vi "formal - Copy (2).vi"() -> ()   [LabVIEW 2011]
uses:
  <vilib>/DAQmx/read.llb/DAQmx Read (Analog 1D Wfm NChan NSamp).vi
  <vilib>/DAQmx/configure/timing.llb/DAQmx Timing (Sample Clock).vi
  <vilib>/DAQmx/miscellaneous.llb/DAQmx Fill In Error Info.vi
  C:/Program Files (x86)/National Instruments/LabVIEW 2011/resource/objmgr/daqmx.rc
  <vilib>/Analysis/NI_AALBase.lvlib
panel:
  out "Channel Name Array":string[](array[string])
  in  "index (col)":i32
  in  "voltage excitation source 2":i32(ring)=10200 items=["Internal"=10200, "External"=10167, "None"=10230]
  out "Config Array":T1(array[cluster])=[{[], "Voltage_cluster"={0.0, 0.0, 0.0, 0.0, TRUE, 0.0, 0.0}, "Strain_cluster"={0.0, 0.0, 0.0, 0.0, TRUE, 0.0, 0.0, 0.0, 0.0, ""}}, {[], "Voltage_cluster"={0.0, 0.0, 0.0, 0.0, TRUE, 0.0, 0.0}, "Strain_cluster"={0.0, 0.0, 0.0, 0.0, TRUE, 0.0, 0.0, 0.0, 0.0, ""}}, {[], "Voltage_cluster"={0.0, 0.0, 0.0, 0.0, TRUE, 0.0, 0.0}, "Strain_cluster"={0.0, 0.0, 0.0, 0.0, TRUE, 0.0, 0.0, 0.0, 0.0, ""}}, {[], "Voltage_cluster"={0.0, 0.0, 0.0, 0.0, TRUE, 0.0, 0.0}, "Strain_cluster"={0.0, 0.0, 0.0, 0.0, TRUE, 0.0, 0.0, 0.0, 0.0, ""}}, {[], "Voltage_cluster"={0.0, 0.0, 0.0, 0.0, TRUE, 0.0, 0.0}, "Strain_cluster"={0.0, 0.0, 0.0, 0.0, TRUE, 0.0, 0.0, 0.0, 0.0, ""}}, {[], "Voltage_cluster"={0.0, 0.0, 0.0, 0.0, TRUE, 0.0, 0.0}, "Strain_cluster"={0.0, 0.0, 0.0, 0.0, TRUE, 0.0, 0.0, 0.0, 0.0, ""}}, {[], "Voltage_cluster"={0.0, 0.0, 0.0, 0.0, TRUE, 0.0, 0.0}, "Strain_cluster"={0.0, 0.0, 0.0, 0.0, TRUE, 0.0, 0.0, 0.0, 0.0, ""}}, {[], "Voltage_cluster"={0.0, 0.0, 0.0, 0.0, TRUE, 0.0, 0.0}, "Strain_cluster"={0.0, 0.0, 0.0, 0.0, TRUE, 0.0, 0.0, 0.0, 0.0, ""}}]
  out "LVM result file path":path
  in  "Tab Control":T2(tab)
  out "Utility Usage Array":cluster{bool, string}[][](array[cluster])=[[{TRUE, "hjk"}, {FALSE, ""}, {FALSE, ""}, {FALSE, ""}], [{TRUE, "hjk"}, {FALSE, ""}, {FALSE, ""}, {FALSE, ""}], [{FALSE, ""}, {FALSE, ""}, {FALSE, ""}, {FALSE, ""}], [{FALSE, ""}, {FALSE, ""}, {FALSE, ""}, {FALSE, ""}], [{FALSE, ""}, {FALSE, ""}, {FALSE, ""}, {FALSE, ""}], [{FALSE, ""}, {FALSE, ""}, {FALSE, ""}, {FALSE, ""}], [{FALSE, ""}, {FALSE, ""}, {FALSE, ""}, {FALSE, ""}], [{FALSE, ""}, {FALSE, ""}, {FALSE, ""}, {FALSE, ""}]]
  in  "SXCI Chassis Name":string="/SC1"
  in  "Config File Path":path=path "M:/github/DAQP/xml_temp.xml"
  in  "Task Name":refnum<k21>="new Task"
  in  "Record File Path":string="trial_newnew"
  in  "error in":errorcluster
  in  "custom scale name":tag="linear1"
  in  "voltage excitation source":i32(ring)=10200 items=["Internal"=10200, "External"=10167, "None"=10230]
  in  "error out":errorcluster
  in  "sample rate":dbl=1000.0
  in  "number of samples per channel (buffer size)":i32=10000000
  in  "number of samples per channel":i32=100
  in  "Start DAQ":bool
  out "Result Array":dbl[](graph) caption="Voltage based transducer Reading"
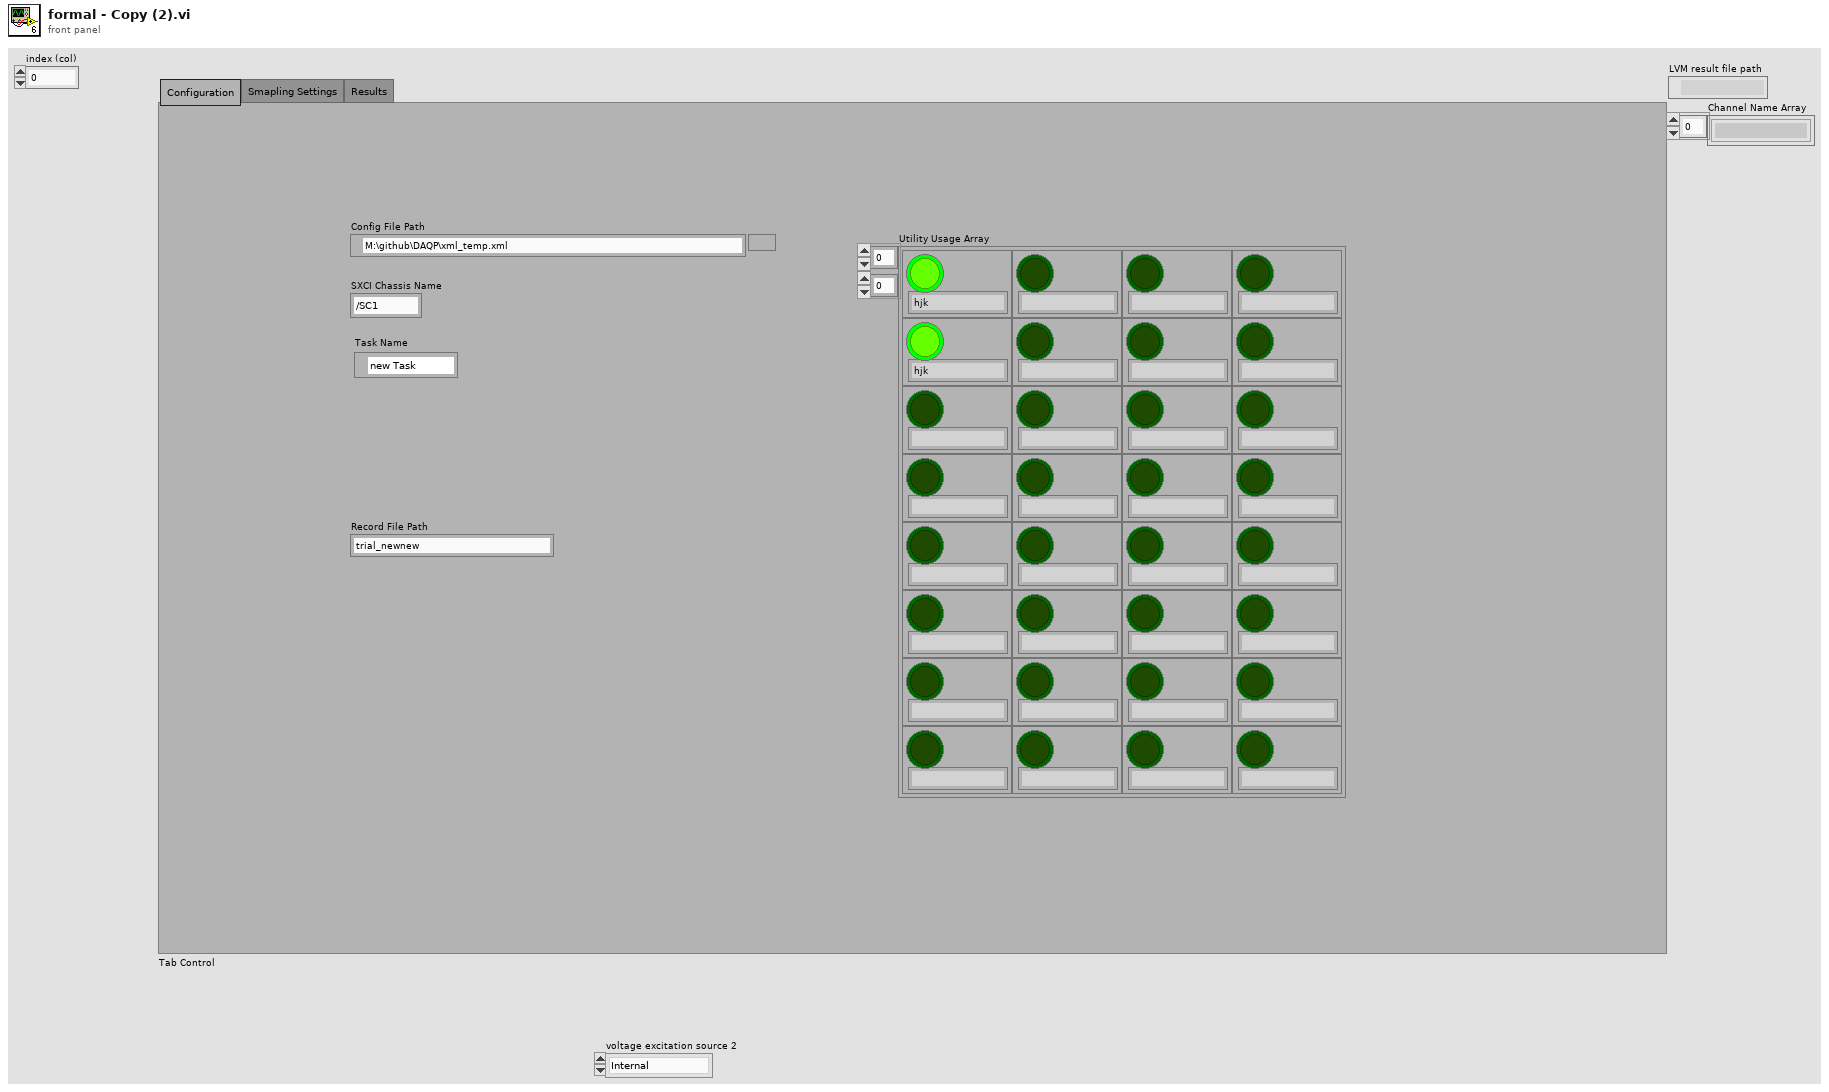
[diagram p1: front panel]
types:
  T1 = cluster{string[], "Voltage_cluster":cluster{dbl, dbl, dbl, dbl, bool, dbl, dbl}, "Strain_cluster":cluster{dbl, dbl, dbl, dbl, bool, dbl, dbl, dbl, dbl, string}}[]
  T2 = enum32{"Configuration", "Smapling Settings", "Results"}
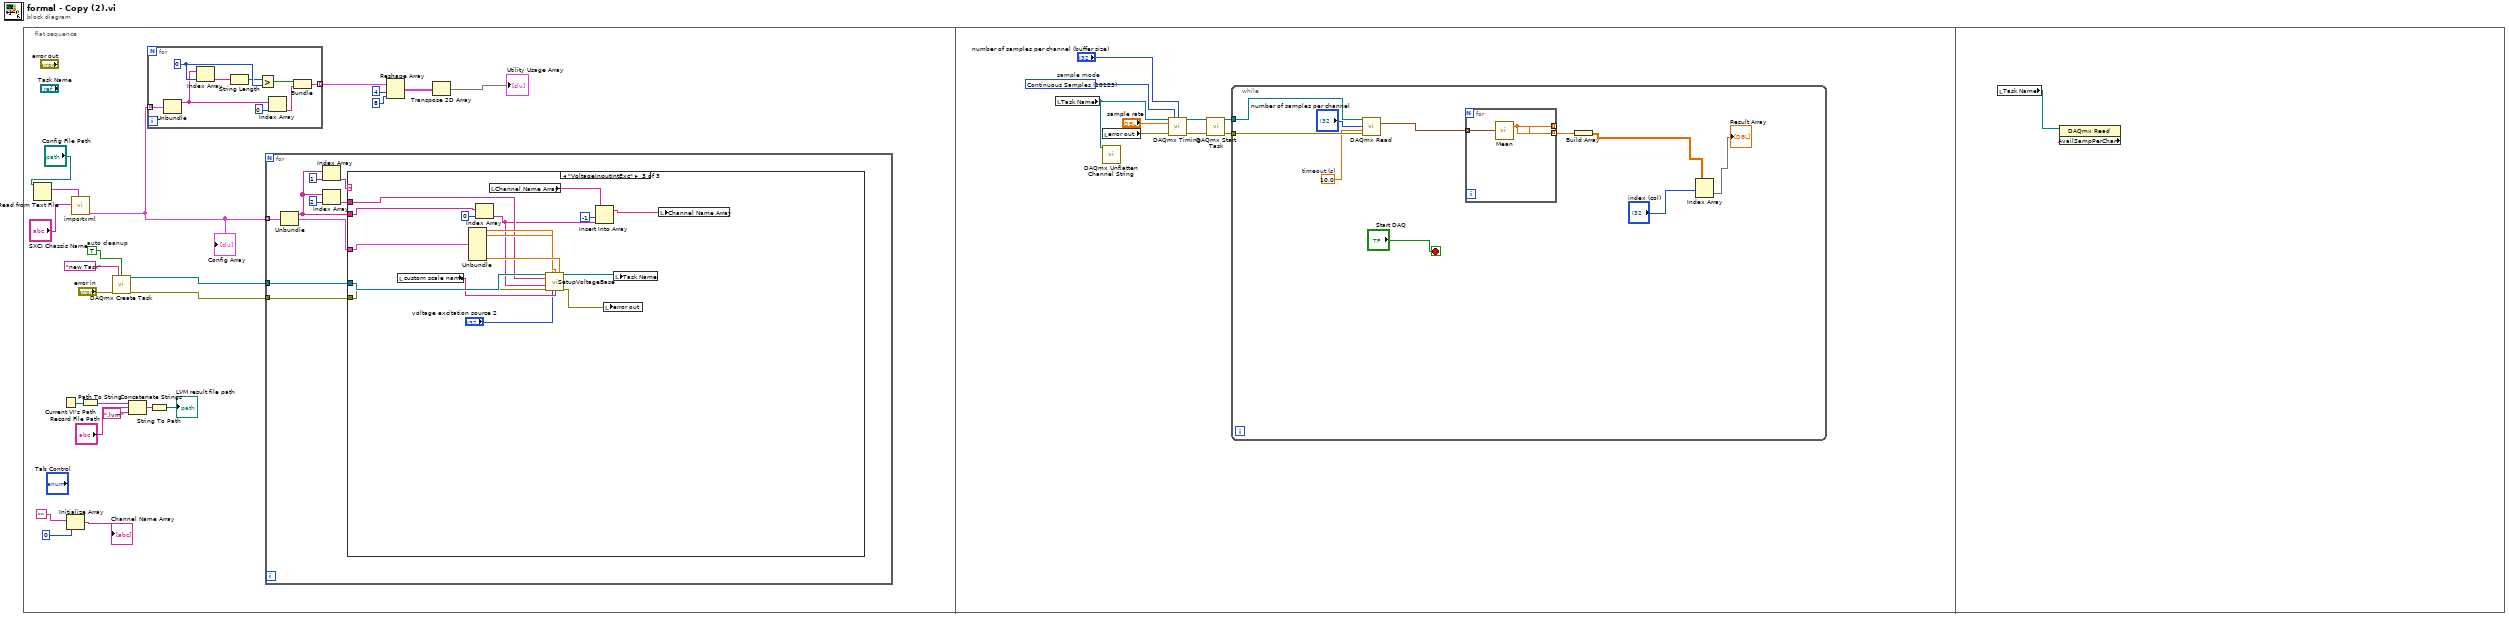
[diagram p0: block diagram]
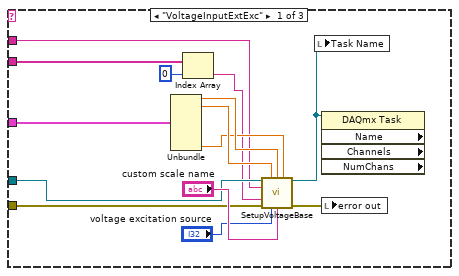
[diagram p2: hidden frame]
diagram:
  n1 = flat-sequence {
    frame #0 {
      w13 = TRUE  # auto cleanup
      n2 = Read from Text File(file (use dialog)="Config File Path") -> (text=w22:string)  [unwired: 3 in, 3 out]
      n3 = Current VI's Path() -> (path=w8:path)
      n4 = Initialize Array("", 0 ("dimension size")) -> (→"Channel Name Array":string[])
      n5 = call "importxml.vi"("String"=w22, "sc"="SXCI Chassis Name") -> ("output array"=w11:T1)  [unwired: 9 in]
      "Config Array" <- w11
      n6 = Path To String(path=w8) -> (string=w9:string)
      n7 = call <vilib>:"DAQmx Create Task.vi"("new task name"="new Task", "auto cleanup"=w13, "error in"="error in") -> ("task out"=w15:refnum<k21>, "error out"=w14:errorcluster)  [unwired: 2 in, 9 out]
      n8 = Concatenate Strings(w9, "Record File Path", ".lvm") -> (w6:string)
      n9 = for {
        tunnel: w11 -> [w72] mode=indexing
        tunnel: [w64] -> w17 mode=indexing
        w70 = 0 ("index")
        n10 = Unbundle(w72) -> (w67:string[])  [unwired: 2 out]
        n11 = Index Array(array=w67, index=w70) -> (element=w71:string)
        n12 = String Length(string=w71) -> (length=w69:i32)
        n13 = Greater?(x=w69, y=w70) -> (0:w66:bool)
        n14 = Index Array(array=w67, index=0) -> (element=w65:string)
        n15 = Bundle(w66, w65) -> (w64:cluster{bool, string})  [unwired: 1 in]
      }
      n16 = String To Path(string=w6) -> (path=→"LVM result file path":path)
      n17 = for {
        tunnel: w11 -> [w32] mode=indexing
        tunnel: w15 -> [w29]
        tunnel: w14 -> [w28]
        n18 = Unbundle(w32) -> (w25:string[], "Voltage_cluster"=w27:cluster{dbl, dbl, dbl, dbl, bool, dbl, dbl})  [unwired: 1 out]
        n19 = Index Array(array=w25, index=1) -> (element=w30:string)
        n20 = Index Array(array=w25, index=2) -> (element=w24:string)
        n21 = case shown="\"VoltageInputIntExc\"" w30 {
          tunnel: w29 -> [w42 _ w61]
          tunnel: w28 -> [w41 _ w60]
          tunnel: w27 -> [w40 _ w62]
          tunnel: w25 -> [w39 _ w59]
          tunnel: w24 -> [w34 _ w50]
          frame "VoltageInputExtExc" {
            n22 = Unbundle(w40) -> (w45:dbl, w44:dbl, w35:dbl)  [unwired: 4 out]
            n23 = Index Array(array=w39, index=0) -> (element=w33:string)
            n24 = call "SetupVoltageBase.vi"("Refnum in"=w42, "Numeric"=w44, "Numeric 2"=w45, "excitation value"=w35, "physical channel"=w34, "String"=w33, "error in (no error)"=w41, "voltage excitation source"="voltage excitation source", "custom scale name"="custom scale name") -> ("Refnum out"=w36:refnum<k21>, "error out"=w37:errorcluster)  [unwired: 5 in]
            n25 = local write "Task Name"(w36) -> ()
            n26 = property class="DAQmx Task" props=["Name", "Channels", "NumChans"](reference=w36) -> ()  [unwired: 1 in, 5 out]
            n27 = local write "error out"(w37) -> ()
          }
          frame "Null", Default {
          }
          frame "VoltageInputIntExc" {
            n28 = local read "custom scale name"() -> (w57:tag)
            n29 = Unbundle(w62) -> (w53:dbl, w52:dbl, w58:dbl)  [unwired: 4 out]
            n30 = Index Array(array=w59, index=0) -> (element=w48:string)
            n31 = local read "Channel Name Array"() -> (w49:string[])
            n32 = call "SetupVoltageBase.vi"("Refnum in"=w61, "Numeric"=w52, "Numeric 2"=w53, "excitation value"=w58, "physical channel"=w50, "String"=w48, "error in (no error)"=w60, "voltage excitation source"="voltage excitation source 2", "custom scale name"=w57) -> ("Refnum out"=w55:refnum<k21>, "error out"=w54:errorcluster)  [unwired: 5 in]
            n33 = Insert Into Array(array=w49, index=-1, new element=w48) -> (w51:string[])
            n34 = local write "error out"(w54) -> ()
            n35 = local write "Task Name"(w55) -> ()
            n36 = local write "Channel Name Array"(w51) -> ()
          }
        }
      }
      n37 = Reshape Array(w17, 4 ("dimension size"), 8 ("dimension size")) -> (w19:cluster{bool, string}[][])
      n38 = Transpose 2D Array(2D array=w19) -> (transposed array=→"Utility Usage Array":cluster{bool, string}[][])
    }
    frame #1 {
      w79 = 10123 items=["Finite Samples"=10178, "Continuous Samples"=10123, "Hardware Timed Single Point"=12522]  # sample mode
      n39 = local read "Task Name"() -> (w76:refnum<k21>)
      n40 = local read "error out"() -> (w75:errorcluster)
      n41 = call <vilib>:"DAQmx Unflatten Channel String.vi"("names in"=w76) -> ()  [unwired: 1 in, 14 out]
      n42 = call-poly <vilib>:"DAQmx Timing.vi"("task/channels in"=w76, "sample mode"=w79, "samples per channel"="number of samples per channel (buffer size)", "rate"="sample rate", "error in"=w75) -> ("task out"=w78:refnum<k21>, "error out"=w77:errorcluster)  [unwired: 2 in, 7 out]
      n43 = call <vilib>:"DAQmx Start Task.vi"("task/channels in"=w78, "error in"=w77) -> ("task out"=w74:refnum<k21>, "error out"=w73:errorcluster)  [unwired: 12 out]
      n44 = while {
        tunnel: w74 -> [w91]
        tunnel: w73 -> [w90]
        stop <- "Start DAQ" stop-if-true
        w87 = 10.0  # timeout (s)
        n45 = call-poly <vilib>:"DAQmx Read.vi"("task/channels in"=w91, "number of samples per channel"="number of samples per channel", "timeout"=w87, "error in"=w90) -> ("data"=w86:waveform(dbl)[])  [unwired: 9 in, 2 out]
        n46 = for {
          tunnel: w86 -> [w92] mode=indexing
          tunnel: [w93] -> _ mode=indexing
          tunnel: [w93] -> w85 mode=indexing
          n47 = call <vilib>:"Mean.vi"("X"=w92) -> ("mean"=w93:dbl)  [unwired: 1 out]
        }
        n48 = Build Array(w85) -> (w83:dbl[][])
        n49 = Index Array(array=w83, index (col)="index (col)") -> (element=→"Result Array":dbl[])  [unwired: 1 in]
      }
    }
    frame #2 {
      n50 = local read "Task Name"() -> (w94:refnum<k21>)
      n51 = property class="DAQmx Read" props=["AvailSampPerChan"](reference=w94) -> ()  [unwired: 1 in, 3 out]
    }
  }
